vi "timer.vi"(7 "pauza":bool, 10 "Czas":dbl) -> (3 "czy czas upłynął":bool)   [LabVIEW 2014]
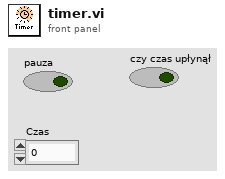
[diagram p1: front panel]
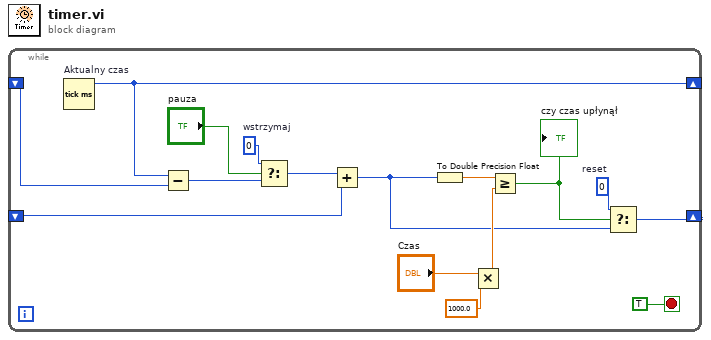
[diagram p0: block diagram]
diagram:
  n1 = while {
    shift-right: [w4] -> _
    shift-left: _ -> [w3]
    shift-right: [w5] -> _
    shift-left: _ -> [w6]
    stop <- TRUE stop-if-true
    w15 = u32 0  # wstrzymaj
    w12 = u32 0  # reset
    n2 = Tick Count (ms) "Aktualny czas"() -> (millisecond timer value=w4:u32)
    n3 = Subtract(x=w4, y=w3) -> (x-y=w14:u32)
    n4 = Select(t=w15, s="pauza", f=w14) -> (s? t:f=w16:u32)
    n5 = Add(x=w16, y=w6) -> (x+y=w2:u32)
    n6 = To Double Precision Float(number=w2) -> (double precision float=w1:dbl)
    n7 = Multiply(x="Czas", y=1000.0) -> (x*y=w11:dbl)
    n8 = Greater Or Equal?(x=w1, y=w11) -> (x >= y?=w13:bool)
    "czy czas upłynął" <- w13
    n9 = Select(t=w12, s=w13, f=w2) -> (s? t:f=w5:u32)
  }
